vi "labview_demo.vi"() -> ()   [LabVIEW 2021]
uses:
  user.lib/CycloneControlSDK/CycloneControlSDK.lvlib
panel:
  in  "Image ID":u32=1
  out "Error Code":i32 format="%x"
  out "Error String":string
  out "Success":bool
  out "Pass Count":u32
  out "Launch":bool
  out "Error":bool
  in  "Port Identifier":string(combo)="USB1"
  in  "Start Button":bool
  out "Connect":bool
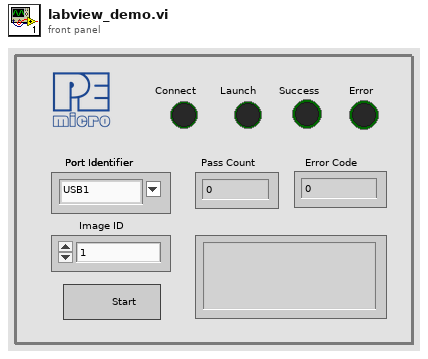
[diagram p1: front panel]
types:
  T1 = enum8{"Enabled", "Disabled", "Disabled and Grayed Out"}
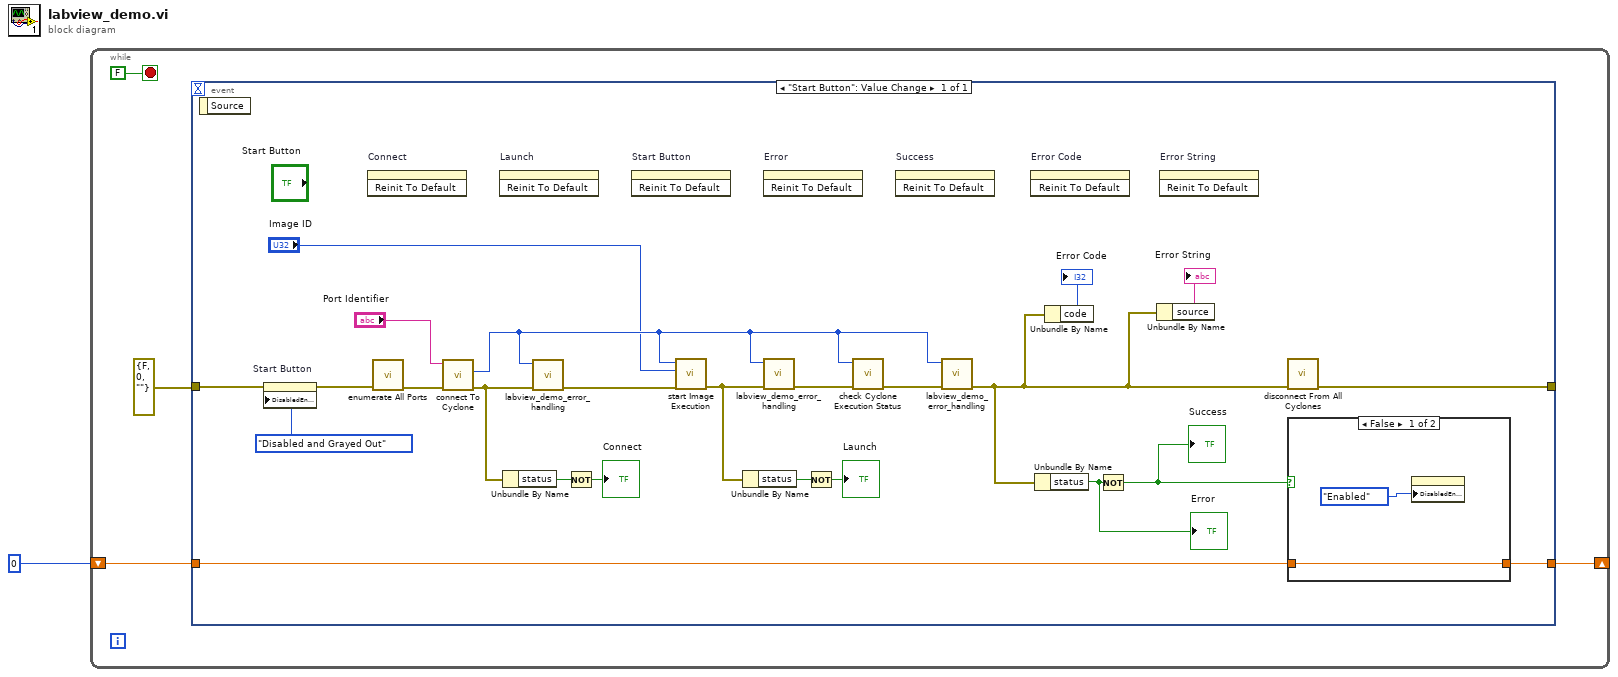
[diagram p0: block diagram]
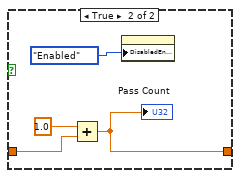
[diagram p2: hidden frame]
diagram:
  n1 = while {
    shift-right: [w4] -> _
    shift-left: 0 -> [w3]
    stop <- FALSE stop-if-true
    n2 = event shown="[0] \"Start Button\": Value Change" {
      selector: _ -> [_]
      dyn-events: _ -> [_]
      timeout: _ -> [_]
      tunnel: [w21] -> w4
      tunnel: w3 -> [w22]
      tunnel: errorcluster {"status"=FALSE, "code"=0, "source"=""} ("error constant") -> [w11]
      tunnel: [w20] -> _
      event "Start Button": Value Change {
        n3 = event-data() -> ()  [unwired: 1 in, 1 out]
        n4 = property on="Start Button" class="Bool"(error in=w11, "DisabledEnum"=T1."Disabled and Grayed Out" ("Disabled")) -> (error out=w10:errorcluster)  [unwired: 1 in, 1 out]
        n5 = invoke on="Connect" class="Bool (strict)" method="Reinit To Default"() -> ()  [unwired: 3 in, 3 out]
        n6 = call "enumerate All Ports.vi"("error in"=w10) -> ("error out"=w29:errorcluster)  [unwired: 10 in]
        n7 = call "connect To Cyclone.vi"("error in"=w29, "nameIpOrPortIdentifier"="Port Identifier") -> ("error out"=w19:errorcluster, "function return"=w8:u32)  [unwired: 7 in, 1 out]
        n8 = invoke on="Launch" class="Bool (strict)" method="Reinit To Default"() -> ()  [unwired: 3 in, 3 out]
        n9 = Unbundle By Name(w19) -> ("status"=w28:bool)
        n10 = call "labview_demo_error_handling.vi"("error in"=w19, "cycloneHandle"=w8) -> ("error out"=w18:errorcluster)  [unwired: 9 in]
        n11 = Not(x=w28) -> (.not. x?=→"Connect":bool)
        n12 = invoke on="Start Button" class="Bool" method="Reinit To Default"() -> ()  [unwired: 3 in, 3 out]
        n13 = call "start Image Execution.vi"("error in"=w18, "imageId"="Image ID", "cycloneHandle"=w8) -> ("error out"=w17:errorcluster)  [unwired: 7 in, 1 out]
        n14 = Unbundle By Name(w17) -> ("status"=w26:bool)
        n15 = invoke on="Error" class="Bool (strict)" method="Reinit To Default"() -> ()  [unwired: 3 in, 3 out]
        n16 = call "labview_demo_error_handling.vi"("error in"=w17, "cycloneHandle"=w8) -> ("error out"=w16:errorcluster)  [unwired: 9 in]
        n17 = Not(x=w26) -> (.not. x?=→"Launch":bool)
        n18 = call "check Cyclone Execution Status.vi"("error in"=w16, "cycloneHandle"=w8) -> ("error out"=w15:errorcluster)  [unwired: 8 in, 1 out]
        n19 = invoke on="Success" class="Bool (strict)" method="Reinit To Default"() -> ()  [unwired: 3 in, 3 out]
        n20 = call "labview_demo_error_handling.vi"("error in"=w15, "cycloneHandle"=w8) -> ("error out"=w13:errorcluster)  [unwired: 9 in]
        n21 = invoke on="Error Code" class="DigNum (strict)" method="Reinit To Default"() -> ()  [unwired: 3 in, 3 out]
        n22 = Unbundle By Name(w13) -> ("status"=w24:bool)
        "Error" <- w24
        n23 = Unbundle By Name(w13) -> ("code"=→"Error Code":i32)
        n24 = Not(x=w24) -> (.not. x?=w23:bool)
        "Success" <- w23
        n25 = Unbundle By Name(w13) -> ("source"=→"Error String":string)
        n26 = invoke on="Error String" class="Str" method="Reinit To Default"() -> ()  [unwired: 3 in, 3 out]
        n27 = call "disconnect From All Cyclones.vi"("error in"=w13) -> ("error out"=w20:errorcluster)  [unwired: 10 in]
        n28 = case shown="False" w23 {
          tunnel: [w31 w35] -> w21
          tunnel: w22 -> [w31 w33]
          frame False {
            n29 = property on="Start Button" class="Bool"("DisabledEnum"=T1."Enabled" ("Disabled")) -> ()  [unwired: 2 in, 2 out]
          }
          frame True {
            n30 = Add(x=1.0 ("y"), y=w33) -> (x+y=w35:dbl)
            "Pass Count" <- w35
            n31 = property on="Start Button" class="Bool"("DisabledEnum"=T1."Enabled" ("Disabled")) -> ()  [unwired: 2 in, 2 out]
          }
        }
      }
    }
  }
